vi "Initialize.vi"(5 "Retry Attempts (0)":i32 min=0, 7 "Serial Configuration":T1={"Baud Rate"=9600, "Parity"=0, "Flow Control"=0, "Data Bits"=8, "Stop Bits"=10} {"Stop Bits" items=["1"=10, "1.5"=15, "2"=20]; "Data Bits" items=["8"=8]; "Flow Control" items=["None", "XON/XOFF", "RTS/CTS", "XON/XOFF & RTS/CTS", "DTR/DSR", "XON/XOFF & DTR/DSR"]; "Parity" items=["None"]; "Baud Rate" items=["9600"=9600, "19200"=19200]}, 8 "error in (no error)":errorcluster, 9 "Reset (True)":bool=TRUE, 10 "ID Query (True)":bool=TRUE, 11 "VISA resource name":refnum<visa-resource-name>="COM1") -> (0 "error out":errorcluster, 2 "Address ID (-1 if ID Query = False)":i32, 3 "VISA resource name out":refnum<visa-resource-name>)   [LabVIEW 2020, in "Omega Platinum Series.lvlib"]
doc: "Establishes communication with the instrument and optionally performs an instrument identification query and/or an instrument reset. It also places the instrument in a default state needed for other instrument driver operations. Therefore, call this VI before calling other instrument driver VIs for this instrument. Generally, you need to call the <b>Initialize</b> VI only once at the beginning of an application."
uses:
  <instrlib>/RxnRover/OmegaPlatinumSeriesDriver/Omega Platinum Series.lvlib
panel:
  # "(c) 2019 <Enter Company Name Here>.  ALL RIGHTS RESERVED."
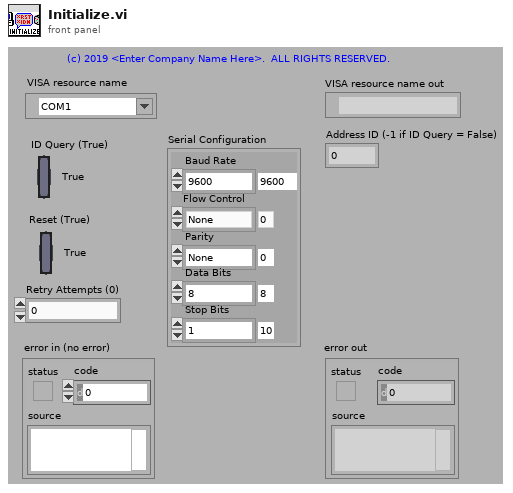
[diagram p1: front panel]
types:
  T1 = cluster{"Baud Rate":u32, "Parity":u16, "Flow Control":u16, "Data Bits":u16, "Stop Bits":u16}
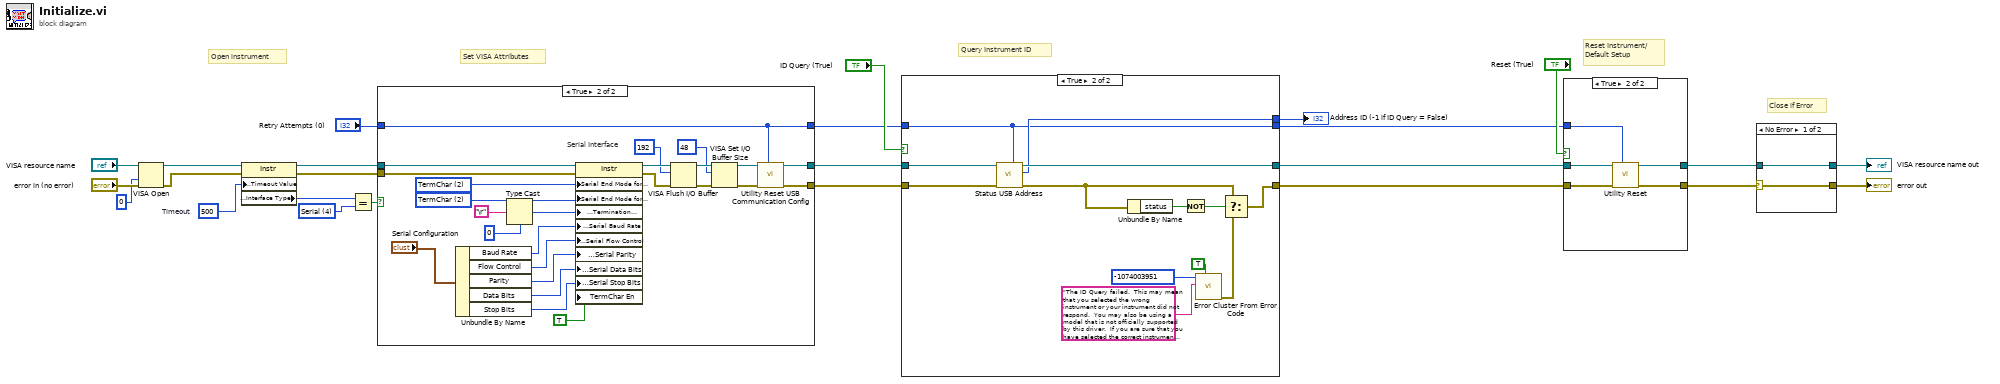
[diagram p0: block diagram]
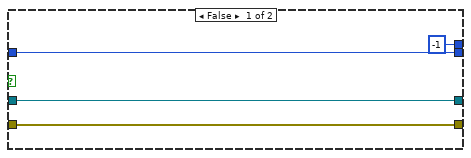
[diagram p3: hidden frame]
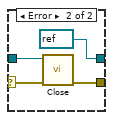
[diagram p5: hidden frame]
diagram:
  w17 = u16 4 items=["GPIB"=1, "VXI"=2, "GPIB-VXI"=3, "Serial"=4, "PXI"=5, "TCPIP"=6, "USB"=7] ("Interface Information:Interface Type")
  w21 = u32 500  # Timeout
  # "Query Instrument ID"
  # "Set VISA Attributes"
  # "Close if Error"
  # "Reset Instrument/\nDefault Setup"
  # "Open instrument"
  n1 = VISA Open(access mode=u32 0, error in (no error)="error in (no error)", VISA resource name="VISA resource name") -> (VISA resource name=w15:refnum<visa-resource-name>, error out=w14:errorcluster)  [unwired: 2 in]
  n2 = property class="Instr"(reference=w15, error in=w14, "General Settings:Timeout Value"=w21) -> (reference out=w20:refnum<visa-resource-name>, error out=w19:errorcluster, "Interface Information:Interface Type"=w22:u16)
  n3 = Equal?(x=w22, y=w17) -> (x = y?=w18:bool)
  n4 = case shown="True" w18 {
    tunnel: [w27 w30] -> w10
    tunnel: [w28 w32] -> w9
    tunnel: w20 -> [w27 w36]
    tunnel: w19 -> [w28 w35]
    tunnel: "Retry Attempts (0)" -> [w26 w29]
    tunnel: [w26 w29] -> w2
    frame False {
      # "EDIT: Remove interfaces not supported by your instrument."
      # "GPIB, TCP/IP, and USB Interface"
    }
    frame True {
      w39 = u16 2 items=["None", "LastBit", "TermChar"] ("Serial Settings:Serial End Mode for Reads")
      w45 = u16 2 items=["None", "LastBit", "TermChar"] ("Serial Settings:Serial End Mode for Reads")
      # "Serial Interface"
      n5 = Unbundle By Name("Serial Configuration") -> ("Baud Rate"=w43:u32, "Flow Control"=w40:u16, "Parity"=w42:u16, "Data Bits"=w38:u16, "Stop Bits"=w37:u16)
      n6 = Type Cast(type=u8 0, x="\r") -> (*(type *) &x=w44:u8)
      n7 = property class="Instr"(reference=w36, error in=w35, "Serial Settings:Serial End Mode for Reads"=w45, "Serial Settings:Serial End Mode for Writes"=w39, "Message Based Settings:Termination Character"=w44, "Serial Settings:Serial Baud Rate"=w43, "Serial Settings:Serial Flow Control"=w40, "Serial Settings:Serial Parity"=w42, "Serial Settings:Serial Data Bits"=w38, "Serial Settings:Serial Stop Bits"=w37, "TermChar En"=TRUE ("Message Based Settings:Termination Character Enable")) -> (reference out=w49:refnum<visa-resource-name>, error out=w52:errorcluster)
      n8 = VISA Flush I/O Buffer(VISA resource name=w49, mask (16)=u16 192, error in (no error)=w52) -> (VISA resource name out=w53:refnum<visa-resource-name>, error out=w51:errorcluster)
      n9 = VISA Set I/O Buffer Size(VISA resource name=w53, mask (16)=u16 48, error in (no error)=w51) -> (VISA resource name out=w31:refnum<visa-resource-name>, error out=w50:errorcluster)  [unwired: 1 in]
      n10 = call <instrlib>:"Utility Reset USB Communication Config.vi"("Retry Attempts (0)"=w29, "error in (no error)"=w50, "VISA resource name (in)"=w31) -> ("error out"=w32:errorcluster, "VISA resource name (out)"=w30:refnum<visa-resource-name>)  [unwired: 6 in, 1 out]
    }
  }
  n11 = case shown="True" "ID Query (True)" {
    tunnel: [w56 w70] -> w8
    tunnel: [w57 w63] -> w7
    tunnel: w10 -> [w57 w69]
    tunnel: w9 -> [w56 w62]
    tunnel: [-1 ("Address") w60] -> w5
    tunnel: w2 -> [w54 w58]
    tunnel: [w54 w58] -> w1
    frame False {
    }
    frame True {
      n12 = call <instrlib>:"Status USB Address.vi"("Retry Attempts (0)"=w58, "error in (no error)"=w62, "VISA resource name (in)"=w69) -> ("error out"=w61:errorcluster, "Address"=w60:i32, "VISA resource name (out)"=w63:refnum<visa-resource-name>)  [unwired: 6 in]
      n13 = Unbundle By Name(w61) -> ("status"=w64:bool)
      n14 = Not(x=w64) -> (.not. x?=w59:bool)
      n15 = call <vilib>:"Error Cluster From Error Code.vi"("show call chain? (False)"=TRUE, "error message (\"\")"="The ID Query failed.  This may mean that you selected the wrong instrument or your instrument did not respond.  You may also be using a model that is not officially supported by this driver.  If you are sure that you have selected the correct instrument and it is responding, try disabling the ID Query." ("Source (VI Name)"), "error code (0)"=-1074003951 ("Code")) -> ("error out"=w68:errorcluster)  [unwired: 6 in]
      n16 = Select(t=w61, s=w59, f=w68) -> (s? t:f=w70:errorcluster)
    }
  }
  "Address ID (-1 if ID Query = False)" <- w5
  n17 = case shown="True" "Reset (True)" {
    tunnel: w8 -> [w71 w77]
    tunnel: [w71 w76] -> w12
    tunnel: w7 -> [w72 w75]
    tunnel: [w72 w74] -> w13
    tunnel: w1 -> [_ w73]
    frame False {
    }
    frame True {
      n18 = call <instrlib>:"Utility Reset.vi"("Retry Attempts (0)"=w73, "error in (no error)"=w77, "VISA resource name"=w75) -> ("error out"=w76:errorcluster, "VISA resource name out"=w74:refnum<visa-resource-name>)  [unwired: 7 in]
    }
  }
  n19 = case shown="No Error" w12 {
    selector: w12 -> [w78 w81]
    tunnel: w13 -> [w79 w82]
    tunnel: [w79 refnum<visa-resource-name> refnum ("VISA resource name out")] -> w6
    tunnel: [w78 w83] -> w4
    frame No Error {
    }
    frame Error {
      n20 = call <instrlib>:"Close.vi"("error in (no error)"=w81, "VISA resource name"=w82) -> ("error out"=w83:errorcluster)  [unwired: 9 in]
    }
  }
  "VISA resource name out" <- w6
  "error out" <- w4
